vi "CMD StartProcessing.vi"(8 "error in (no error)":errorcluster, 10 "StartProcInitParams":T1={"InverterInfo"={"Inverter ID"=""}, "ProcessInitParams"={"MinCurrThreshold"=1.5, "NumPF RdsToAvg"=2, "ESR alarm threshhold (%)"=200.0, "# readings to average"=40}} {"ProcessInitParams"."MinCurrThreshold" format="%.2f"}, 11 "Main in":refnum<class "Main.lvclass">) -> (0 "error out":errorcluster, 3 "Main out":refnum<class "Main.lvclass">)   [LabVIEW 2019, in "Main.lvclass"]
doc: "Developed by Kevin Thompson\nkevin@thompsonengineering.net\n\nCopyright 2018\nThompson Engineering, LLC"
uses:
  Main.lvclass
  DataTypes/AsynCmd_Main--enum.ctl
  DataTypes/InverterInfo--cluster.ctl
  DataTypes/ProcessInitParams--cluster.ctl
  DataTypes/StartProcInitParams--cluster.ctl
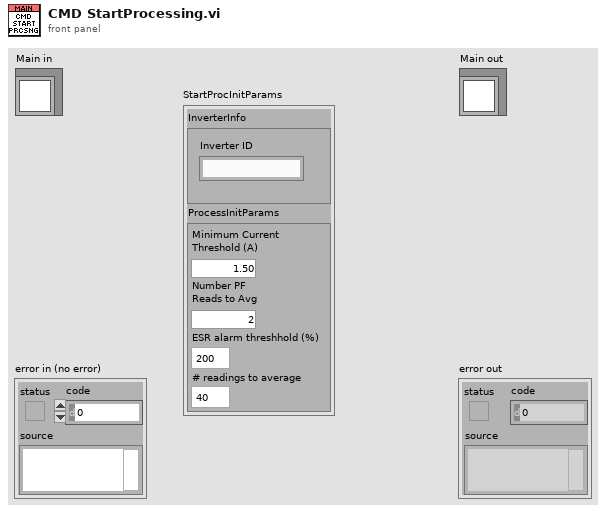
[diagram p1: front panel]
types:
  T1 = typedef "Main.lvclass/StartProcInitParams--cluster.ctl" = cluster{"InverterInfo":T2, "ProcessInitParams":T3}
  T2 = typedef "InverterInfo--cluster.ctl" = cluster{"Inverter ID":string}
  T3 = typedef "Main.lvclass/ProcessInitParams--cluster.ctl" = cluster{"MinCurrThreshold":dbl, "NumPF RdsToAvg":i32, "ESR alarm threshhold (%)":dbl, "# readings to average":i32}
  T4 = typedef "Main.lvclass/AsynCmd_Main--enum.ctl" = enum16{"Main.StartProcessing", "Main.StopProcessing", "Main.RefreshInverterList"}
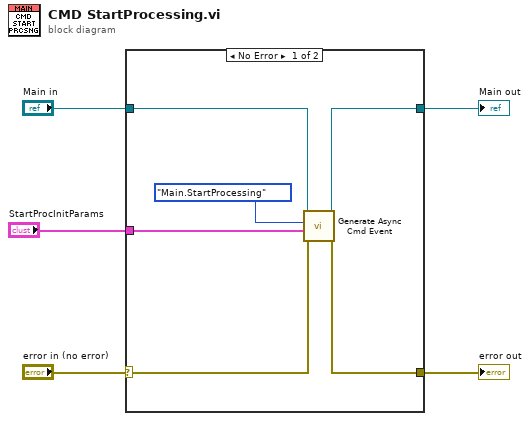
[diagram p0: block diagram]
diagram:
  n1 = case shown="No Error" "error in (no error)" {
    selector: "error in (no error)" -> [w9 w13]
    tunnel: [w8 w13] -> w4
    tunnel: [w10 w12] -> w2
    tunnel: "Main in" -> [w11 w12]
    tunnel: "StartProcInitParams" -> [w6 _]
    frame No Error {
      n2 = call "Generate Async Cmd Event.vi"("error in (no error)"=w9, "vData"=w6, "AsyncCmd"=AsynCmd_Main--enum."Main.StartProcessing", "Main in"=w11) -> ("error out"=w8:errorcluster, "Main out"=w10:refnum<class "Main.lvclass">)  [unwired: 6 in]
    }
    frame Error {
    }
  }
  "error out" <- w4
  "Main out" <- w2
